vi "Progressbar_Get Attributes.vi"(8 "error in (no error)":errorcluster, 11 "Progress In":refnum<class "Progressbar.lvclass">) -> (0 "error out":errorcluster, 2 "Progressbar Attributes":T1, 3 "Progress Out":refnum<class "Progressbar.lvclass">)   [LabVIEW 2017, in "Front Panel Publisher.lvlib" / "Progressbar.lvclass"]
uses:
  Progressbar.lvclass
  Attributes.ctl
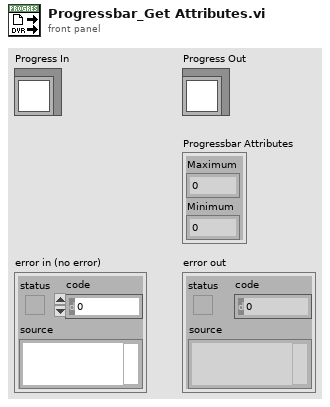
[diagram p1: front panel]
types:
  T1 = typedef "Front Panel Publisher.lvlib/Progressbar.lvclass/Attributes.ctl" = cluster{"Maximum":dbl, "Minimum":dbl}
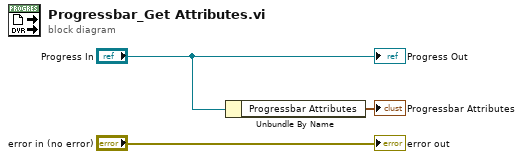
[diagram p0: block diagram]
diagram:
  n1 = Unbundle By Name("Progress In") -> ("Progressbar Attributes"=→"Progressbar Attributes":T1)
  "error out" <- "error in (no error)"
  "Progress Out" <- "Progress In"
